vi "Draw Target Line.vi"(2 "X":dbl, 3 "Image In":T1) -> (1 "Image Out":T1)   [LabVIEW 2013]
uses:
  <vilib>/vision/Image Controls.llb/IMAQ Image.ctl
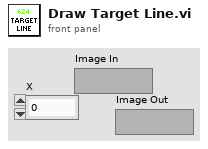
[diagram p1: front panel]
types:
  T1 = typedef "IMAQ Image.ctl" = refnum<image>
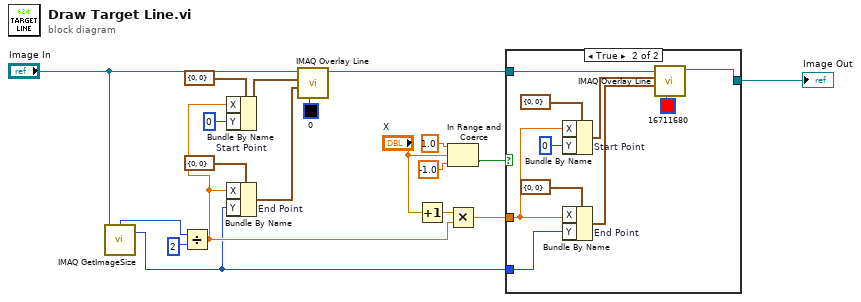
[diagram p0: block diagram]
diagram:
  n1 = call "IMAQ GetImageSize"("Image"="Image In") -> ("Y Resolution"=w1:i32, "X Resolution"=w15:i32)  [unwired: 3 in, 1 out]
  n2 = Divide(x=w15, y=2) -> (x/y=w2:dbl)
  n3 = Bundle By Name "Start Point"(cluster=cluster{"X":i32, "Y":i32} {"X"=0, "Y"=0} ("Start Point"), "X"=w2, "Y"=0) -> (w4:cluster{"X":i32, "Y":i32})
  n4 = Bundle By Name "End Point"(cluster=cluster{"X":i32, "Y":i32} {"X"=0, "Y"=0} ("End Point"), "X"=w2, "Y"=w1) -> (w3:cluster{"X":i32, "Y":i32})
  n5 = call "IMAQ Overlay Line"("Color"=u32 0, "End Point"=w3, "Start Point"=w4, "Image"="Image In") -> ("Image Out"=w9:T1)  [unwired: 6 in, 1 out]
  n6 = Increment(x="X") -> (x+1=w13:dbl)
  n7 = In Range and Coerce(upper limit=1.0, x="X", lower limit=-1.0) -> (In Range?=w18:bool)  [unwired: 1 out]
  n8 = Multiply(x=w13, y=w2) -> (x*y=w11:dbl)
  n9 = case shown="True" w18 {
    tunnel: w11 -> [_ w30]
    tunnel: w9 -> [w20 w24]
    tunnel: [w20 w23] -> w19
    tunnel: w1 -> [_ w21]
    frame False {
    }
    frame True {
      n10 = Bundle By Name "Start Point"(cluster=cluster{"X":i32, "Y":i32} {"X"=0, "Y"=0} ("Start Point"), "X"=w30, "Y"=0) -> (w26:cluster{"X":i32, "Y":i32})
      n11 = Bundle By Name "End Point"(cluster=cluster{"X":i32, "Y":i32} {"X"=0, "Y"=0} ("End Point"), "X"=w30, "Y"=w21) -> (w28:cluster{"X":i32, "Y":i32})
      n12 = call "IMAQ Overlay Line"("Color"=u32 16711680, "End Point"=w28, "Start Point"=w26, "Image"=w24) -> ("Image Out"=w23:T1)  [unwired: 6 in, 1 out]
    }
  }
  "Image Out" <- w19
